vi "ObtainSMQueue.vi"(8 "ErrorArray":errorcluster[](array[cluster]), 10 "BusNumber":i32) -> (0 "ErrorArray":errorcluster[](array[cluster]), 3 "QueRef":T1)   [LabVIEW 2014, in "Bus_class.lvlib" / "Bus.lvclass"]
uses:
  Bus.lvclass
  MsgQueue/Typedef/QueRef.ctl
  MsgQueue/Typedef/MsgQueue.ctl
  SMQueue.ctl
  <userlib>/NIST/NISTErrorLib/NISTErrorLib.lvlib
  Framework.lvlib
panel:
  out "queue name":string
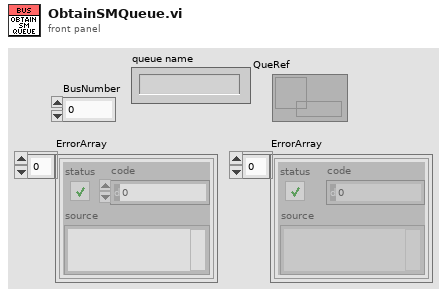
[diagram p1: front panel]
types:
  T1 = typedef "Framework.lvlib/QueRef.ctl" = refnum<queue>
  T2 = typedef "Bus_class.lvlib/Bus.lvclass/SMQueue.ctl" = cluster{"Msg":string, "Data":variant}
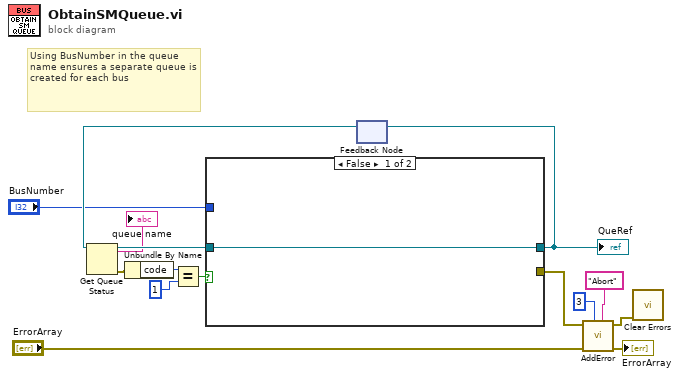
[diagram p0: block diagram]
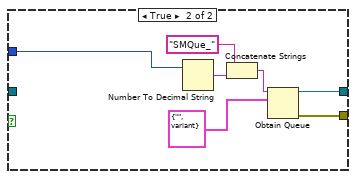
[diagram p2: hidden frame]
diagram:
  # "Using BusNumber in the queue name ensures a separate queue is created for each bus"
  n1 = feedback #1() -> (w14:refnum<queue>)  [unwired: 1 in]
  n2 = Get Queue Status(queue=w14) -> (queue out=w7:refnum<queue>, queue name=→"queue name":string, error out=w6:errorcluster)  [unwired: 2 in, 5 out]
  n3 = Unbundle By Name(w6) -> ("code"=w5:i32)
  n4 = Equal?(x=w5, y=1) -> (x = y?=w8:bool)
  n5 = case shown="False" w8 {
    tunnel: [w16 w23] -> w15
    tunnel: w7 -> [w16 _]
    tunnel: [_ w22] -> w13
    tunnel: "BusNumber" -> [_ w21]
    frame False {
    }
    frame True {
      n6 = Number To Decimal String(number=w21) -> (decimal integer string=w19:string)  [unwired: 1 in]
      n7 = Concatenate Strings("SMQue_" ("name (unnamed)"), w19) -> (w17:string)
      n8 = Obtain Queue(name (unnamed)=w17, element data type=T2 {"Msg"="", "Data"=variant} ("MsgQueue")) -> (queue out=w23:refnum<queue>, error out=w22:errorcluster)  [unwired: 3 in, 1 out]
    }
  }
  "QueRef" <- w15
  n9 = feedback-in #1(w15) -> ()
  n10 = call <userlib>:"AddError.vi"("Severity"="Abort", "Priority"=u8 3, "ErrorArray"="ErrorArray", "error in (no error)"=w13) -> ("ErrorArray"=→"ErrorArray":errorcluster[], "error out"=w2:errorcluster)  [unwired: 6 in]
  n11 = call <vilib>:"Clear Errors.vi"("error in (no error)"=w2) -> ()  [unwired: 5 in, 2 out]
